vi "Read Display-tab.vi"(8 "error in (no error)":errorcluster, 11 "CV-UI in":refnum<class "CV-UI.lvclass">) -> (0 "error out":errorcluster, 2 "Display-tab":refnum<notifier>, 3 "CV-UI out":refnum<class "CV-UI.lvclass">)   [LabVIEW 2013, in "CameraVision.lvlib" / "CV-UI.lvclass"]
uses:
  CV-UI.lvclass
  CV-UI.lvclass/CV-UI.ctl
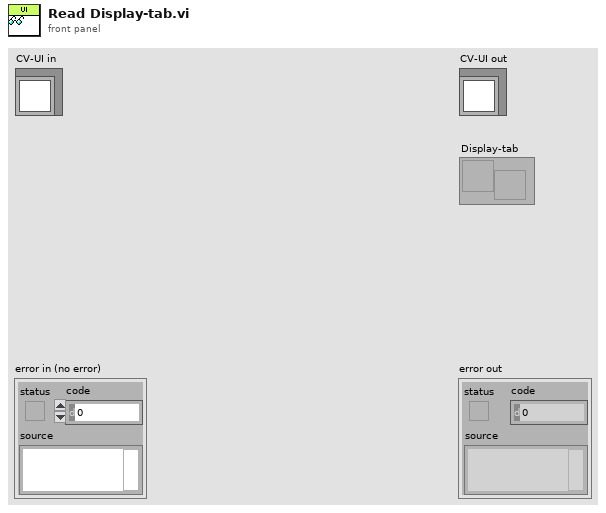
[diagram p1: front panel]
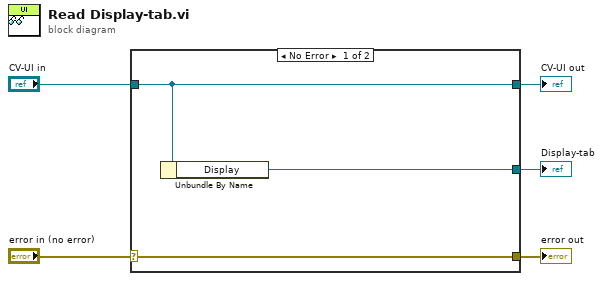
[diagram p0: block diagram]
diagram:
  n1 = case shown="No Error" "error in (no error)" {
    selector: "error in (no error)" -> [w8 w9]
    tunnel: [w8 w9] -> w4
    tunnel: [w7 w10] -> w2
    tunnel: "CV-UI in" -> [w7 w10]
    tunnel: [w6 _] -> w1
    frame No Error {
      n2 = Unbundle By Name(w7) -> ("Display"=w6:refnum<notifier>)
    }
    frame Error {
    }
  }
  "error out" <- w4
  "CV-UI out" <- w2
  "Display-tab" <- w1
